vi "BikeDemo.vi"() -> ()   [LabVIEW 2009]
doc: "Demonstrates the Bike class.\n\nwww.sciware.com.au"
uses:
  Bike/Bike.lvclass
  Racer/Racer.lvclass
panel:
  out "Speed":dbl[](array[numeric])
  in  "Peddle Rate":dbl[](array[numeric])=[2.0, 3.0]
  in  "Gear":i32=2
  # "Bike"
  # "Bike"
  # "Racer"
  # "Racer"
  # "Racer"
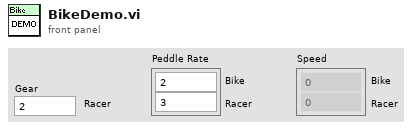
[diagram p1: front panel]
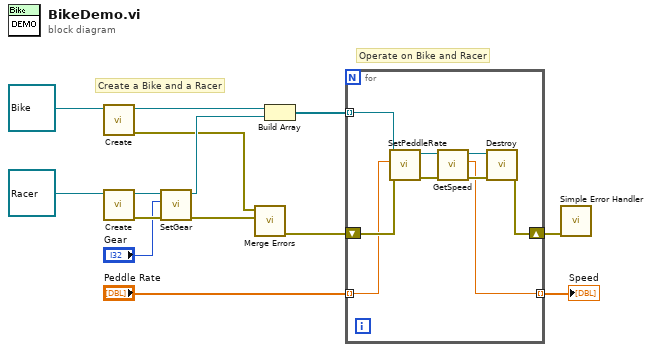
[diagram p0: block diagram]
diagram:
  # "Operate on Bike and Racer"
  # "Create a Bike and a Racer"
  n1 = call-dynamic "Create.vi"("obj"=refnum<class "Bike.lvclass"> refnum) -> ("error out"=w6:errorcluster, "obj out"=w8:refnum<class "Bike.lvclass">)  [unwired: 9 in]
  n2 = call-dynamic "Create.vi"("obj"=refnum<class "Racer.lvclass"> refnum) -> ("error out"=w12:errorcluster, "obj out"=w11:refnum<class "Racer.lvclass">)  [unwired: 9 in]
  n3 = call-dynamic "SetGear.vi"("error in (no error)"=w12, "gear"="Gear", "Bike in"=w11) -> ("error out"=w7:errorcluster, "Bike out"=w9:refnum<class "Racer.lvclass">)  [unwired: 7 in]
  n4 = call <vilib>:"Merge Errors.vi"("error in 2 (no error)"=w7, "error in 1 (no error)"=w6) -> ("error out"=w5:errorcluster)  [unwired: 5 in]
  n5 = Build Array(w8, w9) -> (w4:refnum<class "Bike.lvclass">[])
  n6 = for {
    shift-right: [w17] -> w1
    shift-left: w5 -> [w22]
    tunnel: w4 -> [w23] mode=indexing
    tunnel: "Peddle Rate" -> [w16] mode=indexing
    tunnel: [w15] -> w2 mode=indexing
    n7 = call-dynamic "SetPeddleRate.vi"("error in (no error)"=w22, "peddle rate"=w16, "Bike in"=w23) -> ("error out"=w20:errorcluster, "Bike out"=w21:refnum<class "Bike.lvclass">)  [unwired: 7 in]
    n8 = call-dynamic "GetSpeed.vi"("error in (no error)"=w20, "Bike in"=w21) -> ("error out"=w19:errorcluster, "speed"=w15:dbl, "Bike out"=w18:refnum<class "Bike.lvclass">)  [unwired: 7 in]
    n9 = call-dynamic "Destroy.vi"("error in (no error)"=w19, "obj"=w18) -> ("error out"=w17:errorcluster)  [unwired: 9 in]
  }
  "Speed" <- w2
  n10 = call <vilib>:"Simple Error Handler.vi"("error in (no error)"=w1) -> ()  [unwired: 4 in, 5 out]
